vi "ResetPosition.vi"(8 "error in":errorcluster, 11 "class data in":refnum<class "Sprite.lvclass">) -> (0 "error out":errorcluster, 3 "class data out":refnum<class "Sprite.lvclass">)   [LabVIEW 2010, in "RenderBase.lvlib" / "Sprite.lvclass"]
doc: "Resets the sprite's position to its initial value."
uses:
  Sprite.lvclass
  SceneObject_class/properties/InitialPosition/GetInitialPosition.vi
  SceneObject_class/SceneObject.lvclass
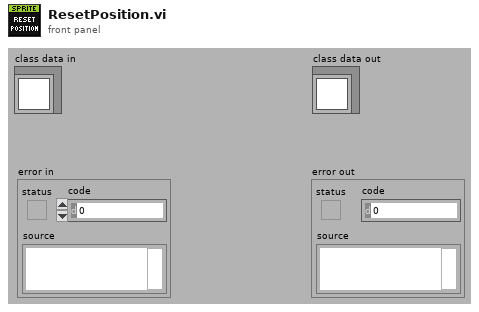
[diagram p1: front panel]
types:
  T1 = typedef "LV3DPointTypeDef.ctl" = cluster{"X":sgl, "Y":sgl, "Z":sgl}
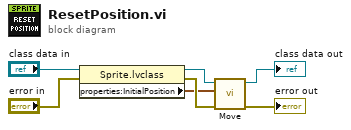
[diagram p0: block diagram]
diagram:
  n1 = property class="Sprite.lvclass"(reference="class data in", error in="error in") -> (reference out=w2:refnum<class "Sprite.lvclass">, error out=w4:errorcluster, "properties:InitialPosition"=w1:T1)
  n2 = call-dynamic "Move.vi"("error in (no error)"=w4, "targetCoords in"=w1, "class data in"=w2) -> ("error out"=→"error out":errorcluster, "class data out"=→"class data out":refnum<class "Sprite.lvclass">)  [unwired: 7 in]
